vi "Get Clicked Cell.vi"(8 "error in (no error)":errorcluster caption="错误输入（无错误）", 11 "Table Ref In":refnum<vi>) -> (0 "error out":errorcluster caption="错误输出", 2 "Clicked Cell":T1, 3 "Table Ref Out":refnum<vi>)   [LabVIEW 2013, in "Table Tool.lvlib"]
uses:
  Table Tool.lvlib
  <vilib>/Utility/miscctls.llb/LVRowAndColumnTypeDef.ctl
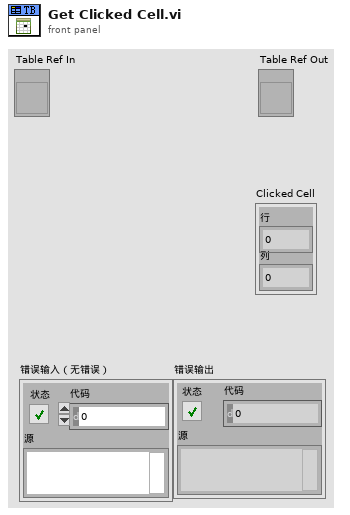
[diagram p1: front panel]
types:
  T1 = typedef "LVRowAndColumnTypeDef.ctl" = cluster{"Row":i32, "Column":i32}
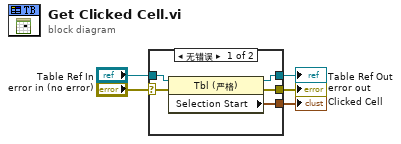
[diagram p0: block diagram]
diagram:
  n1 = case shown="无错误" "error in (no error)" {
    selector: "error in (no error)" -> [w9 w12]
    tunnel: "Table Ref In" -> [w10 w11]
    tunnel: [w7 w11] -> w3
    tunnel: [w8 w12] -> w2
    tunnel: [w6 _] -> w1
    frame No Error {
      n2 = property class="Tbl (严格)"(reference=w10, error in=w9) -> (reference out=w7:refnum<vi>, error out=w8:errorcluster, "Selection Start"=w6:T1)
    }
    frame Error {
    }
  }
  "Table Ref Out" <- w3
  "error out" <- w2
  "Clicked Cell" <- w1
